vi "Write Sonde Data cells to excel.vi"(0 "NI_report in":refnum<class "NI_report.lvclass">, 2 "all rows":string[][](array[string]), 3 "Row Offset In":i32=14, 5 "error in (no error)":errorcluster, 6 "Worksheet Names":string[](array[string]), 7 "Sample Array":i32[](array[numeric]), 9 "Sample Row \nBreak points":i32[](array[numeric]), 11 "Number of Sample Sheets":i32) -> (14 "NI_report out":refnum<class "NI_report.lvclass">, 16 "Row Offset Out":i32, 19 "error out":errorcluster)   [LabVIEW 2016]
uses:
  <vilib>/Utility/NIReport.llb/NI_report.lvclass
panel:
  out "Row Offset":i32
  out "sample subarray":string[][](array[string])
  out "Length":i32
  out "Breakpoint size":i32
  out "number of rows":i32
  out "size(s)":i32[](array[numeric])
  out "Current Sample Sheet":string
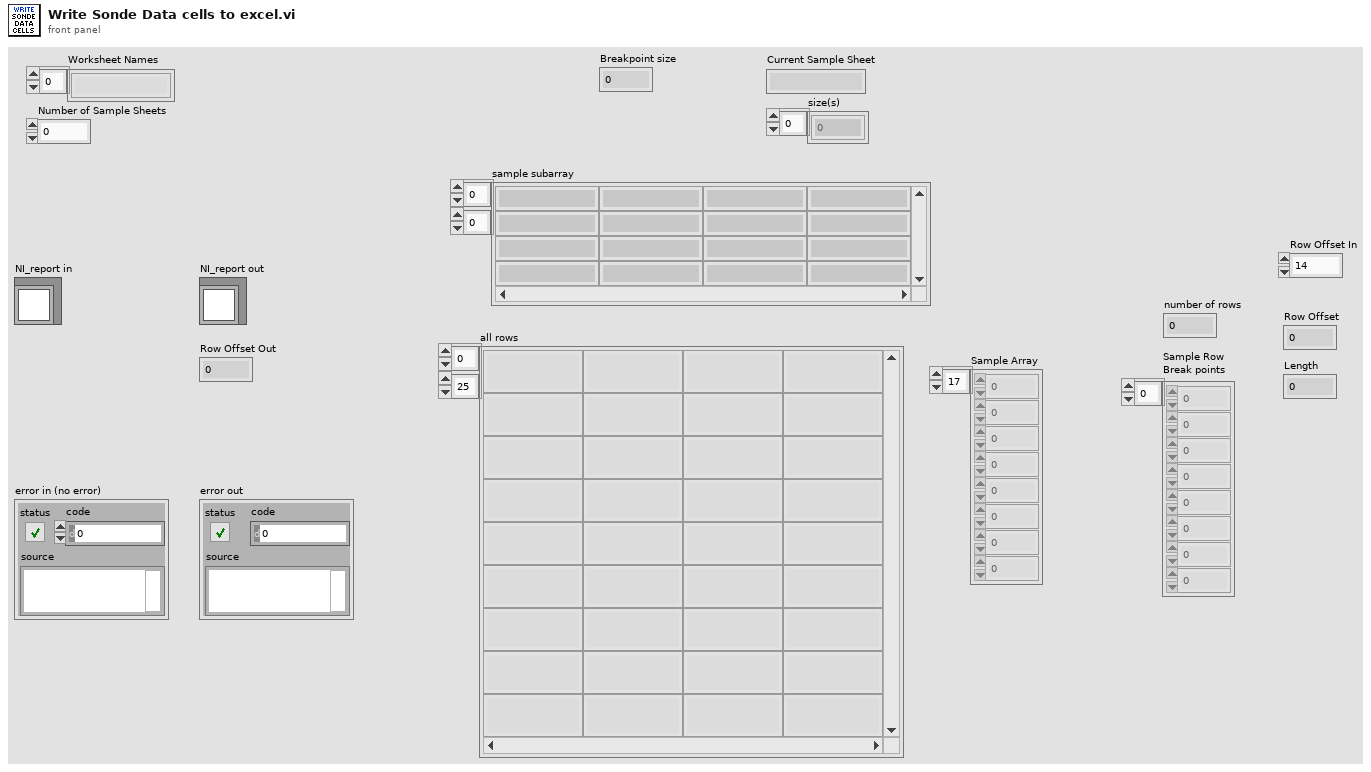
[diagram p1: front panel]
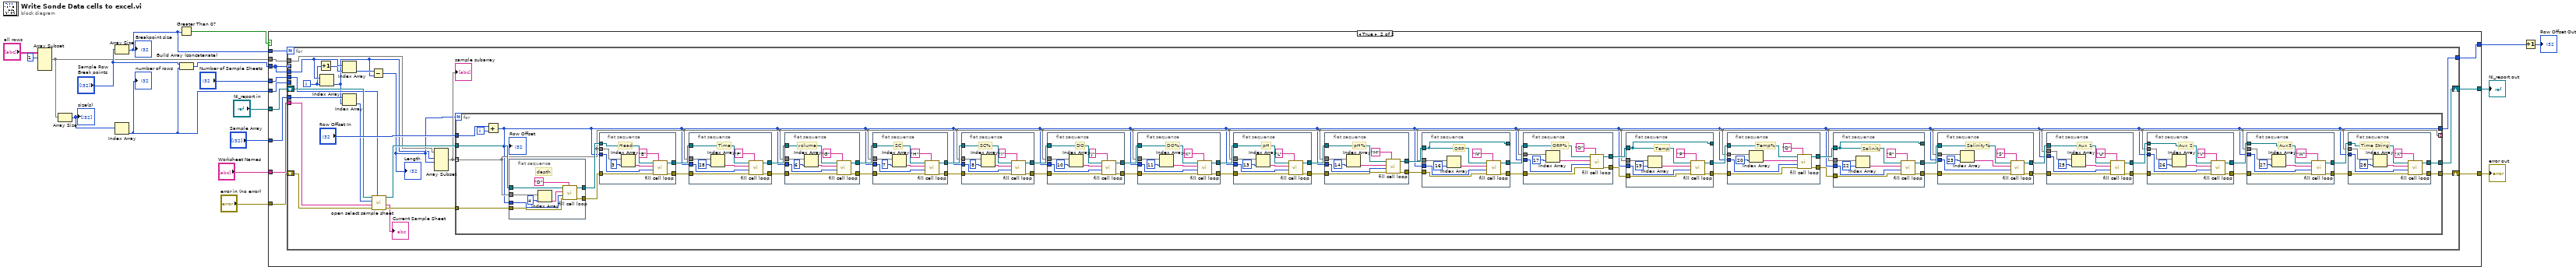
[diagram p0: block diagram]
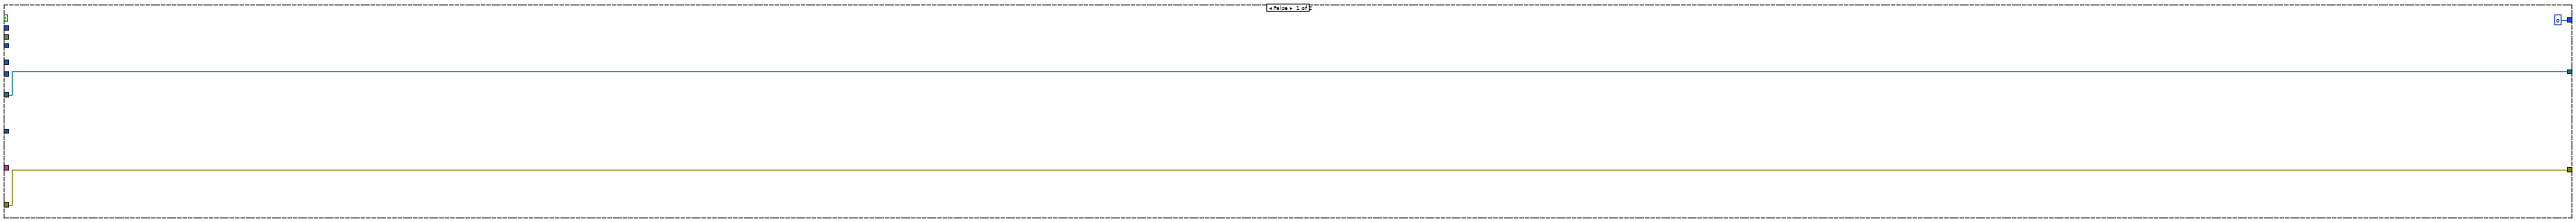
[diagram p2: hidden frame]
diagram:
  n1 = Array Subset(array="all rows", index (row)=1 ("index")) -> (w4:string[][])  [unwired: 3 in]
  n2 = Array Size(array=w4) -> (size(s)=w3:i32[])
  "size(s)" <- w3
  n3 = Array Size(array="Sample Row \nBreak points") -> (size(s)=w11:i32)
  "Breakpoint size" <- w11
  n4 = Index Array(array=w3) -> (element=w1:i32)  [unwired: 1 in]
  "number of rows" <- w1
  n5 = Greater Than 0?(x=w11) -> (x > 0?=w12:bool)
  n6 = Build Array (concatenate)("Sample Row \nBreak points", w1) -> (w2:i32[])
  n7 = case shown="True" w12 {
    tunnel: [w20 w33] -> w18
    tunnel: [w21 w32] -> w17
    tunnel: [0 ("Row Offset In") w31] -> w16
    tunnel: "NI_report in" -> [w21 w30]
    tunnel: "error in (no error)" -> [w20 w29]
    tunnel: w11 -> [_ w28]
    tunnel: w2 -> [_ w23]
    tunnel: "Sample Array" -> [_ w22]
    tunnel: "Worksheet Names" -> [_ w27]
    tunnel: "Number of Sample Sheets" -> [_ w26]
    tunnel: w4 -> [_ w25]
    tunnel: w1 -> [_ w24]
    frame False {
    }
    frame True {
      n8 = for {
        N: w28 -> [_]
        tunnel: [w52] -> w31
        shift-right: [w53] -> w32
        shift-left: w30 -> [w50]
        shift-right: [w54] -> w33
        shift-left: w29 -> [w48]
        tunnel: w23 -> [_] mode=indexing
        tunnel: w23 -> [w43]
        tunnel: w27 -> [w46]
        tunnel: w26 -> [w45]
        tunnel: w25 -> [w40]
        tunnel: w24 -> [_]
        tunnel: w22 -> [w38]
        i -> [w35]
        n9 = Increment(x=w35) -> (x+1=w42:i32)
        n10 = Index Array(array=w43, index=w35) -> (element=w34:i32)
        n11 = Index Array(array=w43, index=w42) -> (element=w39:i32)
        n12 = Index Array(array=w38, index=w34) -> (element=w37:i32)
        n13 = Subtract(x=w39, y=w34) -> (x-y=w36:i32)
        "Length" <- w36
        n14 = call "open select sample sheet.vi"("Number of Sample Sheets"=w45, "error in (no error)"=w48, "Worksheet Names"=w46, "input 1"=w37, "NI_report in"=w50) -> ("error out"=w47:errorcluster, "Current Sample Sheet"=→"Current Sample Sheet":string, "NI_report out"=w49:refnum<class "NI_report.lvclass">)  [unwired: 4 in]
        n15 = Array Subset(array=w40, index (row)=w34, length (row)=w36) -> (w41:string[][])  [unwired: 2 in]
        "sample subarray" <- w41
        n16 = for {
          N: w36 -> [_]
          tunnel: w41 -> [w56] mode=indexing
          tunnel: w49 -> [w96]
          tunnel: w47 -> [w98]
          tunnel: [w58] -> w54
          tunnel: [w57] -> w53
          tunnel: [w56] -> _ mode=indexing
          tunnel: "Row Offset In" -> [w100]
          tunnel: [w55] -> w52
          i -> [w99]
          n17 = Add(x=w100, y=w99) -> (x+y=w55:i32)
          "Row Offset" <- w55
          n18 = flat-sequence {
            tunnel: w56 -> [w279]
            tunnel: w98 -> [w278]
            tunnel: [w277] -> w97
            tunnel: w55 -> [w276]
            tunnel: w96 -> [w274]
            tunnel: [w273] -> w95
            frame #0 {
              # "depth"
              n19 = Index Array(array=w279, index=4) -> (element=w275:string)
              n20 = call "fill cell loop.vi"("Column Letter"="D" ("Depth Column Letter"), "error in (no error)"=w278, "Row"=w276, "String"=w275, "NI_report in"=w274) -> ("error out"=w277:errorcluster, "NI_report out"=w273:refnum<class "NI_report.lvclass">)  [unwired: 5 in]
            }
          }
          n21 = flat-sequence {
            tunnel: [w271] -> w93
            tunnel: [w270] -> w94
            tunnel: w56 -> [w266]
            tunnel: w97 -> [w265]
            tunnel: w55 -> [w264]
            tunnel: w95 -> [w263]
            frame #0 {
              # "Head"
              n22 = Index Array(array=w266, index=3) -> (element=w267:string)
              n23 = call "fill cell loop.vi"("Column Letter"="E" ("Head Column Letter"), "error in (no error)"=w265, "Row"=w264, "String"=w267, "NI_report in"=w263) -> ("error out"=w271:errorcluster, "NI_report out"=w270:refnum<class "NI_report.lvclass">)  [unwired: 5 in]
            }
          }
          n24 = flat-sequence {
            tunnel: [w262] -> w91
            tunnel: [w261] -> w92
            tunnel: w56 -> [w257]
            tunnel: w93 -> [w256]
            tunnel: w55 -> [w255]
            tunnel: w94 -> [w254]
            frame #0 {
              # "Time"
              n25 = Index Array(array=w257, index=28) -> (element=w258:string)
              n26 = call "fill cell loop.vi"("Column Letter"="F" ("Head Column Letter"), "error in (no error)"=w256, "Row"=w255, "String"=w258, "NI_report in"=w254) -> ("error out"=w262:errorcluster, "NI_report out"=w261:refnum<class "NI_report.lvclass">)  [unwired: 5 in]
            }
          }
          n27 = flat-sequence {
            tunnel: [w253] -> w89
            tunnel: [w252] -> w90
            tunnel: w56 -> [w248]
            tunnel: w91 -> [w247]
            tunnel: w55 -> [w246]
            tunnel: w92 -> [w245]
            frame #0 {
              # "volume"
              n28 = Index Array(array=w248, index=6) -> (element=w249:string)
              n29 = call "fill cell loop.vi"("Column Letter"="G" ("Head Column Letter"), "error in (no error)"=w247, "Row"=w246, "String"=w249, "NI_report in"=w245) -> ("error out"=w253:errorcluster, "NI_report out"=w252:refnum<class "NI_report.lvclass">)  [unwired: 5 in]
            }
          }
          n30 = flat-sequence {
            tunnel: [w244] -> w87
            tunnel: [w243] -> w88
            tunnel: w56 -> [w239]
            tunnel: w89 -> [w238]
            tunnel: w55 -> [w237]
            tunnel: w90 -> [w236]
            frame #0 {
              # "SC"
              n31 = Index Array(array=w239, index=7) -> (element=w240:string)
              n32 = call "fill cell loop.vi"("Column Letter"="H" ("Head Column Letter"), "error in (no error)"=w238, "Row"=w237, "String"=w240, "NI_report in"=w236) -> ("error out"=w244:errorcluster, "NI_report out"=w243:refnum<class "NI_report.lvclass">)  [unwired: 5 in]
            }
          }
          n33 = flat-sequence {
            tunnel: [w235] -> w83
            tunnel: [w234] -> w84
            tunnel: w56 -> [w230]
            tunnel: w87 -> [w229]
            tunnel: w55 -> [w228]
            tunnel: w88 -> [w227]
            frame #0 {
              # "SC%"
              n34 = Index Array(array=w230, index=8) -> (element=w231:string)
              n35 = call "fill cell loop.vi"("Column Letter"="I" ("Head Column Letter"), "error in (no error)"=w229, "Row"=w228, "String"=w231, "NI_report in"=w227) -> ("error out"=w235:errorcluster, "NI_report out"=w234:refnum<class "NI_report.lvclass">)  [unwired: 5 in]
            }
          }
          n36 = flat-sequence {
            tunnel: [w226] -> w86
            tunnel: [w225] -> w85
            tunnel: w56 -> [w221]
            tunnel: w83 -> [w220]
            tunnel: w55 -> [w219]
            tunnel: w84 -> [w218]
            frame #0 {
              # "DO"
              n37 = Index Array(array=w221, index=10) -> (element=w222:string)
              n38 = call "fill cell loop.vi"("Column Letter"="J" ("Head Column Letter"), "error in (no error)"=w220, "Row"=w219, "String"=w222, "NI_report in"=w218) -> ("error out"=w226:errorcluster, "NI_report out"=w225:refnum<class "NI_report.lvclass">)  [unwired: 5 in]
            }
          }
          n39 = flat-sequence {
            tunnel: [w217] -> w79
            tunnel: [w216] -> w80
            tunnel: w56 -> [w212]
            tunnel: w86 -> [w211]
            tunnel: w55 -> [w210]
            tunnel: w85 -> [w209]
            frame #0 {
              # "DO%"
              n40 = Index Array(array=w212, index=11) -> (element=w213:string)
              n41 = call "fill cell loop.vi"("Column Letter"="K" ("Head Column Letter"), "error in (no error)"=w211, "Row"=w210, "String"=w213, "NI_report in"=w209) -> ("error out"=w217:errorcluster, "NI_report out"=w216:refnum<class "NI_report.lvclass">)  [unwired: 5 in]
            }
          }
          n42 = flat-sequence {
            tunnel: [w208] -> w81
            tunnel: [w207] -> w82
            tunnel: w56 -> [w203]
            tunnel: w79 -> [w202]
            tunnel: w55 -> [w201]
            tunnel: w80 -> [w200]
            frame #0 {
              # "pH"
              n43 = Index Array(array=w203, index=13) -> (element=w204:string)
              n44 = call "fill cell loop.vi"("Column Letter"="L" ("Head Column Letter"), "error in (no error)"=w202, "Row"=w201, "String"=w204, "NI_report in"=w200) -> ("error out"=w208:errorcluster, "NI_report out"=w207:refnum<class "NI_report.lvclass">)  [unwired: 5 in]
            }
          }
          n45 = flat-sequence {
            tunnel: [w199] -> w76
            tunnel: [w198] -> w75
            tunnel: w56 -> [w194]
            tunnel: w81 -> [w193]
            tunnel: w55 -> [w192]
            tunnel: w82 -> [w191]
            frame #0 {
              # "pH%"
              n46 = Index Array(array=w194, index=14) -> (element=w195:string)
              n47 = call "fill cell loop.vi"("Column Letter"="M" ("Head Column Letter"), "error in (no error)"=w193, "Row"=w192, "String"=w195, "NI_report in"=w191) -> ("error out"=w199:errorcluster, "NI_report out"=w198:refnum<class "NI_report.lvclass">)  [unwired: 5 in]
            }
          }
          n48 = flat-sequence {
            tunnel: [w190] -> w78
            tunnel: [w189] -> w77
            tunnel: w56 -> [w185]
            tunnel: w76 -> [w184]
            tunnel: w55 -> [w183]
            tunnel: [w182] -> _
            tunnel: w75 -> [w182]
            frame #0 {
              # "ORP"
              n49 = Index Array(array=w185, index=16) -> (element=w186:string)
              n50 = call "fill cell loop.vi"("Column Letter"="N" ("Head Column Letter"), "error in (no error)"=w184, "Row"=w183, "String"=w186, "NI_report in"=w182) -> ("error out"=w190:errorcluster, "NI_report out"=w189:refnum<class "NI_report.lvclass">)  [unwired: 5 in]
            }
          }
          n51 = flat-sequence {
            tunnel: [w181] -> w72
            tunnel: [w180] -> w71
            tunnel: w56 -> [w176]
            tunnel: w78 -> [w175]
            tunnel: w55 -> [w174]
            tunnel: w77 -> [w173]
            frame #0 {
              # "ORP%"
              n52 = Index Array(array=w176, index=17) -> (element=w177:string)
              n53 = call "fill cell loop.vi"("Column Letter"="O" ("Head Column Letter"), "error in (no error)"=w175, "Row"=w174, "String"=w177, "NI_report in"=w173) -> ("error out"=w181:errorcluster, "NI_report out"=w180:refnum<class "NI_report.lvclass">)  [unwired: 5 in]
            }
          }
          n54 = flat-sequence {
            tunnel: [w154] -> w68
            tunnel: [w153] -> w67
            tunnel: w56 -> [w149]
            tunnel: w72 -> [w148]
            tunnel: w55 -> [w147]
            tunnel: w71 -> [w146]
            tunnel: [w146] -> _
            frame #0 {
              # "Temp"
              n55 = Index Array(array=w149, index=19) -> (element=w150:string)
              n56 = call "fill cell loop.vi"("Column Letter"="P" ("Head Column Letter"), "error in (no error)"=w148, "Row"=w147, "String"=w150, "NI_report in"=w146) -> ("error out"=w154:errorcluster, "NI_report out"=w153:refnum<class "NI_report.lvclass">)  [unwired: 5 in]
            }
          }
          n57 = flat-sequence {
            tunnel: [w145] -> w69
            tunnel: [w144] -> w70
            tunnel: w56 -> [w140]
            tunnel: w55 -> [w139]
            tunnel: w68 -> [w138]
            tunnel: w67 -> [w137]
            frame #0 {
              # "Temp%"
              n58 = Index Array(array=w140, index=20) -> (element=w141:string)
              n59 = call "fill cell loop.vi"("Column Letter"="Q" ("Head Column Letter"), "error in (no error)"=w138, "Row"=w139, "String"=w141, "NI_report in"=w137) -> ("error out"=w145:errorcluster, "NI_report out"=w144:refnum<class "NI_report.lvclass">)  [unwired: 5 in]
            }
          }
          n60 = flat-sequence {
            tunnel: [w172] -> w73
            tunnel: [w171] -> w74
            tunnel: w56 -> [w167]
            tunnel: w69 -> [w166]
            tunnel: w55 -> [w165]
            tunnel: w70 -> [w164]
            tunnel: [w164] -> _
            frame #0 {
              # "Salinity"
              n61 = Index Array(array=w167, index=22) -> (element=w168:string)
              n62 = call "fill cell loop.vi"("Column Letter"="R" ("Head Column Letter"), "error in (no error)"=w166, "Row"=w165, "String"=w168, "NI_report in"=w164) -> ("error out"=w172:errorcluster, "NI_report out"=w171:refnum<class "NI_report.lvclass">)  [unwired: 5 in]
            }
          }
          n63 = flat-sequence {
            tunnel: [w163] -> w65
            tunnel: [w162] -> w66
            tunnel: w56 -> [w158]
            tunnel: w73 -> [w157]
            tunnel: w55 -> [w156]
            tunnel: w74 -> [w155]
            frame #0 {
              # "Salinity%"
              n64 = Index Array(array=w158, index=23) -> (element=w159:string)
              n65 = call "fill cell loop.vi"("Column Letter"="S" ("Head Column Letter"), "error in (no error)"=w157, "Row"=w156, "String"=w159, "NI_report in"=w155) -> ("error out"=w163:errorcluster, "NI_report out"=w162:refnum<class "NI_report.lvclass">)  [unwired: 5 in]
            }
          }
          n66 = flat-sequence {
            tunnel: [w136] -> w63
            tunnel: [w135] -> w64
            tunnel: w56 -> [w131]
            tunnel: w65 -> [w130]
            tunnel: w55 -> [w129]
            tunnel: w66 -> [w128]
            frame #0 {
              # "Aux 1"
              n67 = Index Array(array=w131, index=25) -> (element=w132:string)
              n68 = call "fill cell loop.vi"("Column Letter"="U" ("Head Column Letter"), "error in (no error)"=w130, "Row"=w129, "String"=w132, "NI_report in"=w128) -> ("error out"=w136:errorcluster, "NI_report out"=w135:refnum<class "NI_report.lvclass">)  [unwired: 5 in]
            }
          }
          n69 = flat-sequence {
            tunnel: [w127] -> w62
            tunnel: [w126] -> w61
            tunnel: w56 -> [w122]
            tunnel: w63 -> [w121]
            tunnel: w55 -> [w120]
            tunnel: w64 -> [w119]
            frame #0 {
              # "Aux 2"
              n70 = Index Array(array=w122, index=26) -> (element=w123:string)
              n71 = call "fill cell loop.vi"("Column Letter"="V" ("Head Column Letter"), "error in (no error)"=w121, "Row"=w120, "String"=w123, "NI_report in"=w119) -> ("error out"=w127:errorcluster, "NI_report out"=w126:refnum<class "NI_report.lvclass">)  [unwired: 5 in]
            }
          }
          n72 = flat-sequence {
            tunnel: [w118] -> w59
            tunnel: [w117] -> w60
            tunnel: w56 -> [w113]
            tunnel: w62 -> [w112]
            tunnel: w55 -> [w111]
            tunnel: w61 -> [w110]
            frame #0 {
              # "Aux3"
              n73 = Index Array(array=w113, index=27) -> (element=w114:string)
              n74 = call "fill cell loop.vi"("Column Letter"="W" ("Head Column Letter"), "error in (no error)"=w112, "Row"=w111, "String"=w114, "NI_report in"=w110) -> ("error out"=w118:errorcluster, "NI_report out"=w117:refnum<class "NI_report.lvclass">)  [unwired: 5 in]
            }
          }
          n75 = flat-sequence {
            tunnel: [w109] -> w58
            tunnel: [w108] -> w57
            tunnel: w56 -> [w104]
            tunnel: w59 -> [w103]
            tunnel: w55 -> [w102]
            tunnel: w60 -> [w101]
            frame #0 {
              # "Time String"
              n76 = Index Array(array=w104, index=28) -> (element=w105:string)
              n77 = call "fill cell loop.vi"("Column Letter"="X" ("Head Column Letter"), "error in (no error)"=w103, "Row"=w102, "String"=w105, "NI_report in"=w101) -> ("error out"=w109:errorcluster, "NI_report out"=w108:refnum<class "NI_report.lvclass">)  [unwired: 5 in]
            }
          }
        }
      }
    }
  }
  "error out" <- w18
  "NI_report out" <- w17
  n78 = Increment(x=w16) -> (x+1=→"Row Offset Out":i32)
